vi "LMS_SendStream.vi"(6 "meta":T2, 7 "samples":dbl[](array[numeric]), 8 "error in (no error)":errorcluster, 9 "timeout_ms":u64, 10 "stream":T1, 11 "sample_count":u64) -> (0 "error out":errorcluster, 3 "return":i32)   [LabVIEW 2018, in "LMS_LV_Drv.lvlib"]
uses:
  LMS_LV_Drv.lvlib
  Stream_ctl.ctl
  C:/Program Files/PothosSDR/bin/LimeSuite.dll
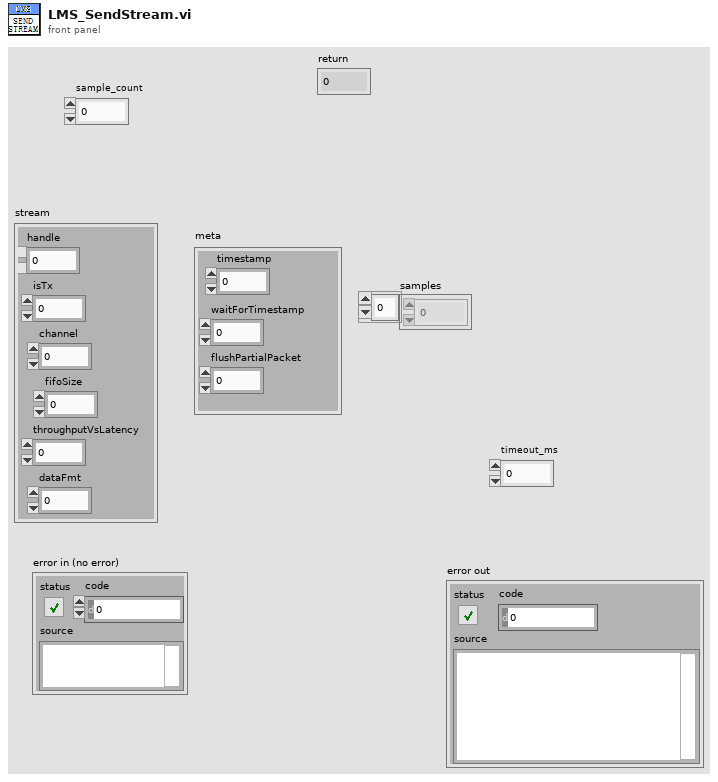
[diagram p1: front panel]
types:
  T1 = typedef "Stream_ctl.ctl" = cluster{"handle":u64, "isTx":u8, "channel":u32, "fifoSize":u32, "throughputVsLatency":dbl, "dataFmt":u32}
  T2 = cluster{"timestamp":u64, "waitForTimestamp":u8, "flushPartialPacket":u8}
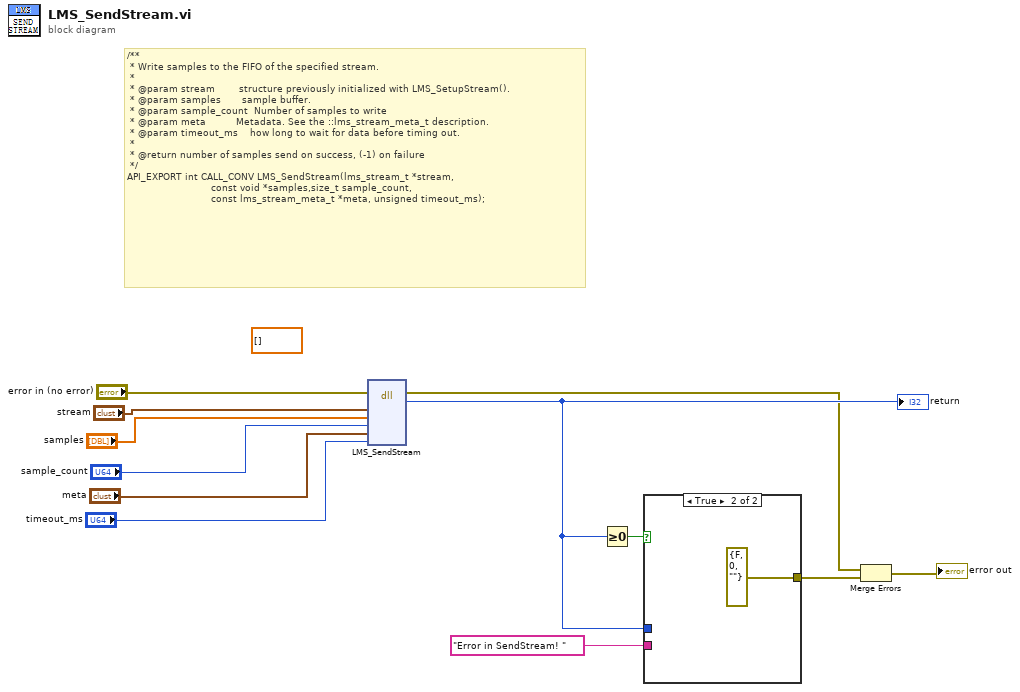
[diagram p0: block diagram]
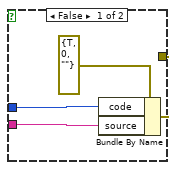
[diagram p2: hidden frame]
diagram:
  (unwired) sgl[] [] ("samples")
  # "/**\n * Write samples to the FIFO of the specified stream.\n *\n * @param stream        structure previously initialized with LMS_SetupStream().\n * @param samples       sample buffer.\n * @param sample_count  Number of samples to write\n * @param meta          Metadata. See the ::lms_stream_meta_t description.\n * @param timeout_ms    how long to wait for data before timing out.\n *\n * @return number of samples send on success, (-1) on failure\n */\nAPI_EXPORT int CALL_CONV LMS_SendStream(lms_stream_t *stream,\n                            const void *samples,size_t sample_count,\n                            const lms_stream_meta_t *meta, unsigned timeout_ms);"
  n1 = dll-call lib="C:/Program Files/PothosSDR/bin/LimeSuite.dll" fn="LMS_SendStream"(error in="error in (no error)", "steam"="stream", "samples"="samples", "sample_count"="sample_count", "meta"="meta", "timeout_ms"="timeout_ms") -> (error out=w3:errorcluster, "return type"=w4:i32)  [unwired: 7 in, 1 out]
  "return" <- w4
  n2 = Greater Or Equal To 0?(x=w4) -> (x >= 0?=w7:bool)
  n3 = case shown="True" w7 {
    tunnel: [w15 errorcluster {"status"=FALSE, "code"=0, "source"=""} ("error in")] -> w5
    tunnel: w4 -> [w14 _]
    tunnel: "Error in SendStream! " ("source") -> [w13 _]
    frame False {
      n4 = Bundle By Name(cluster=errorcluster {"status"=TRUE, "code"=0, "source"=""} ("error in"), "code"=w14, "source"=w13) -> (w15:errorcluster)
    }
    frame True {
    }
  }
  n5 = Merge Errors(w3, w5) -> (→"error out":errorcluster)
